vi "Insert table - 2.vi"() -> ()   [LabVIEW 2015]
uses:
  <vilib>/Platform/TimedLoop/XDataNode/timing_clust.ctl
  <vilib>/Platform/TimedLoop/XDataNode/nitl_modes.ctl
  <vilib>/Platform/TimedLoop/XDataNode/wakeup.ctl
  <vilib>/addons/database/Connection.llb/DB Tools Open Connec (Path).vi
  <vilib>/platform/TimedLoop/XDataNode/XDataNode.xnode
  <vilib>/addons/database/NI_Database_API.lvlib
  <vilib>/Platform/TimedLoop/XDataNode/XDNodeRunTimeDep.lvlib
panel:
  out "floor(x/y)":dbl
  out "Time":u32
  out "Counter":i32
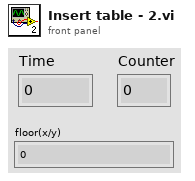
[diagram p1: front panel]
types:
  T1 = typedef "NI_Database_API.lvlib/Conn ObjectReference.ctl" = refnum<k1>
  T2 = typedef "XDNodeRunTimeDep.lvlib/timing_clust.ctl" = cluster{"Expected End [f-1]":u64, "Actual End [f-1]":u64, "Finished Late? [f-1]":bool, "Expected End [i-1]":u64, "Actual End [i-1]":u64, "Finished Late? [i-1]":bool, "Expected Start [i]":u64, "Actual Start [i]":u64, "Expected Start [f]":u64, "Actual Start [f]":u64, "Source Name":string, "Structure Name":string, "Period":i64, "Deadline":i64, "Offset":i64, "Start":i64, "Priority":i32, "Timeout":i32, "Mode":T3, "Wakeup Reason":T4, "Error":errorcluster, "Source Type":string, "Secondary Source Type":string, "Global End Time":u64, "Global Start Time":u64, "Frame Duration":u64, "Iteration Duration":u64, "Assigned CPU":i32, "I/O Scan Engine Mode":u32}
  T3 = typedef "XDNodeRunTimeDep.lvlib/nitl_modes.ctl" = enum32{"No Change", "Process missed periods, maintain original phase", "Discard missed periods, maintain original phase", "Process missed periods, ignore original phase", "Discard missed periods, ignore original phase"}
  T4 = typedef "XDNodeRunTimeDep.lvlib/wakeup.ctl" = enum32{"Normal", "Aborted", "Asynchronous wakeup", "Timing source error", "Timed loop error", "Timeout"}
  T5 = cluster{i32, i32, i32, i32, i32, i32, i32, i32, i32, i32, i32, i32, i32, i32, i32, i32, i32, i32, i32, i32, i32, i32, i32, i32, i32, i32, i32, i32, i32, i32, i32, i32, i32, i32, i32, i32, i32, i32, i32, i32, i32, i32, i32, i32, i32, i32, i32, i32, i32, i32, i32, i32, i32, i32, i32, i32, i32, i32, i32, i32, i32, i32, i32, i32, i32, i32, i32, i32, i32, i32, i32, i32, i32, i32, i32, i32, i32, i32, i32, i32, i32, i32, i32, i32, i32, i32, i32, i32, i32, i32, i32, i32, i32, i32, i32, i32, i32, i32, i32, i32}
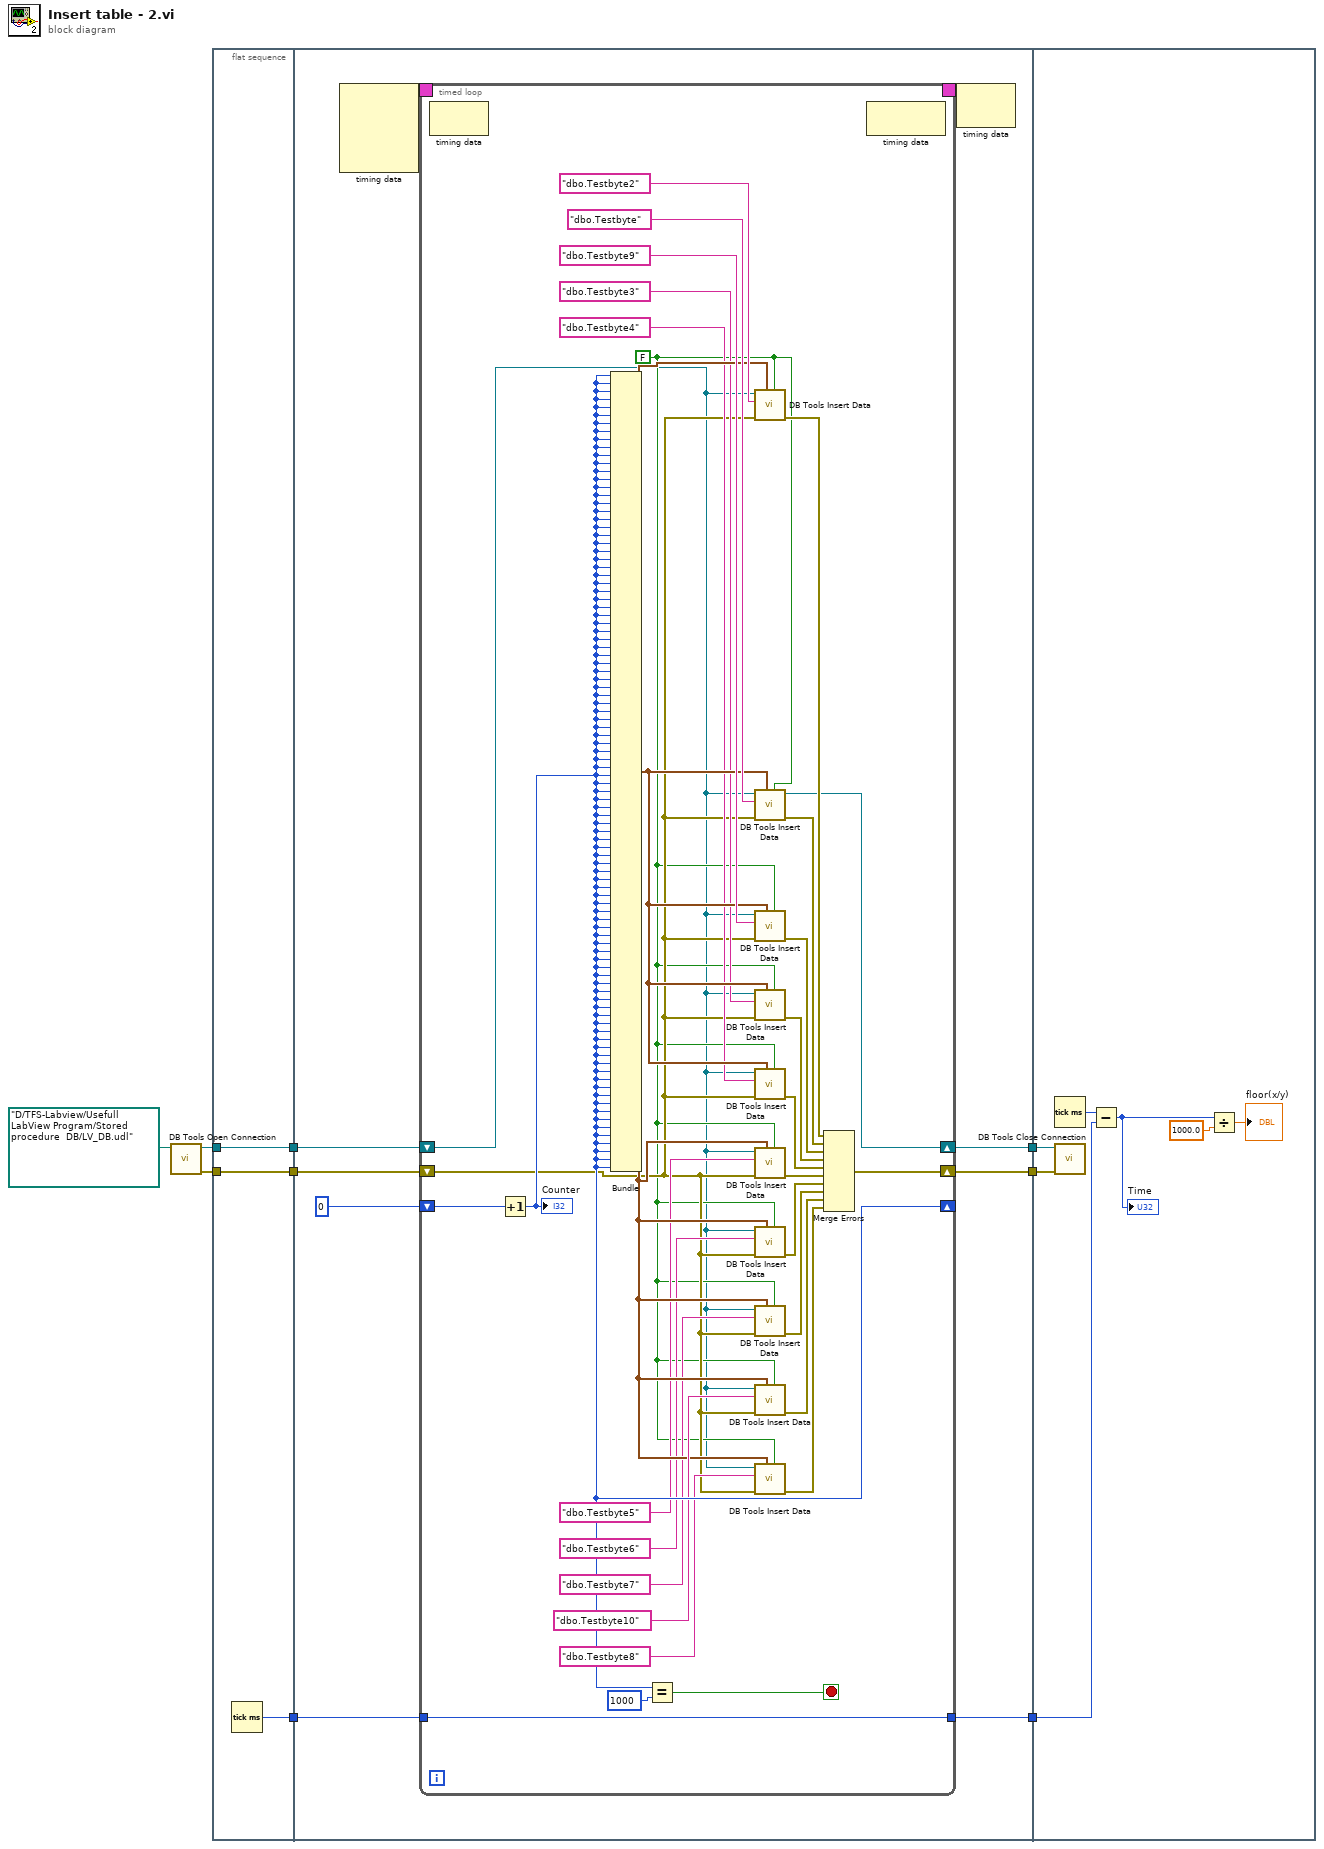
[diagram p0: block diagram]
diagram:
  n1 = call-poly <vilib>:"DB Tools Open Connection.vi"("connection information"=path "D:/TFS-Labview/Usefull LabView Program/Stored procedure  DB/LV_DB.udl") -> ("error out"=w1:errorcluster, "connection reference"=w3:T1)  [unwired: 7 in]
  n2 = flat-sequence {
    tunnel: [w12] -> w9
    tunnel: [w11] -> w8
    tunnel: w3 -> [w11]
    tunnel: [w10] -> w2
    tunnel: w1 -> [w10]
    tunnel: [w20] -> w7
    tunnel: [w18] -> w6
    tunnel: w9 -> [w19]
    tunnel: w8 -> [w17]
    tunnel: [w16] -> w5
    tunnel: w2 -> [w15]
    tunnel: w7 -> [w60]
    tunnel: w6 -> [w62]
    tunnel: w5 -> [w61]
    frame #0 {
      n3 = Tick Count (ms)() -> (millisecond timer value=w12:u32)
    }
    frame #1 {
      n4 = node-c288() -> (w14:T2)  [unwired: 4 in]
      n5 = timed-loop {
        shift-right: [w44] -> w20
        shift-left: w15 -> [w33]
        shift-right: [w43] -> _
        shift-left: 0 -> [w52]
        tunnel: [w51] -> w18
        tunnel: w19 -> [w51]
        shift-right: [w23] -> w16
        shift-left: w17 -> [w22]
        timing: w14 -> [_]
        timing-out: [_] -> w13
        stop <- w49 stop-if-true
        w24 = FALSE ("create table? (F)")
        n6 = node-c288() -> ()  [unwired: 1 in, 1 out]
        n7 = Increment(x=w52) -> (x+1=w43:i32)
        "Counter" <- w43
        n8 = Bundle(w43, w43, w43, w43, w43, w43, w43, w43, w43, w43, w43, w43, w43, w43, w43, w43, w43, w43, w43, w43, w43, w43, w43, w43, w43, w43, w43, w43, w43, w43, w43, w43, w43, w43, w43, w43, w43, w43, w43, w43, w43, w43, w43, w43, w43, w43, w43, w43, w43, w43, w43, w43, w43, w43, w43, w43, w43, w43, w43, w43, w43, w43, w43, w43, w43, w43, w43, w43, w43, w43, w43, w43, w43, w43, w43, w43, w43, w43, w43, w43, w43, w43, w43, w43, w43, w43, w43, w43, w43, w43, w43, w43, w43, w43, w43, w43, w43, w43, w43, w43) -> (w39:T5)  [unwired: 1 in]
        n9 = Equal?(x=w43, y=1000 ("Numeric")) -> (x = y?=w49:bool)
        n10 = call <vilib>:"DB Tools Insert Data.vi"("create table? (F)"=w24, "data"=w39, "error in (no error)"=w33, "table"="dbo.Testbyte2" ("SQL query"), "connection reference"=w22) -> ("error out"=w46:errorcluster)  [unwired: 5 in, 1 out]
        n11 = call <vilib>:"DB Tools Insert Data.vi"("create table? (F)"=w24, "data"=w39, "error in (no error)"=w33, "table"="dbo.Testbyte" ("SQL query"), "connection reference"=w22) -> ("error out"=w45:errorcluster, "connection reference out"=w23:T1)  [unwired: 5 in]
        n12 = call <vilib>:"DB Tools Insert Data.vi"("create table? (F)"=w24, "data"=w39, "error in (no error)"=w33, "table"="dbo.Testbyte9" ("SQL query"), "connection reference"=w22) -> ("error out"=w32:errorcluster)  [unwired: 5 in, 1 out]
        n13 = call <vilib>:"DB Tools Insert Data.vi"("create table? (F)"=w24, "data"=w39, "error in (no error)"=w33, "table"="dbo.Testbyte3" ("SQL query"), "connection reference"=w22) -> ("error out"=w31:errorcluster)  [unwired: 5 in, 1 out]
        n14 = call <vilib>:"DB Tools Insert Data.vi"("create table? (F)"=w24, "data"=w39, "error in (no error)"=w33, "table"="dbo.Testbyte4" ("SQL query"), "connection reference"=w22) -> ("error out"=w30:errorcluster)  [unwired: 5 in, 1 out]
        n15 = call <vilib>:"DB Tools Insert Data.vi"("create table? (F)"=w24, "data"=w39, "error in (no error)"=w33, "table"="dbo.Testbyte5" ("SQL query"), "connection reference"=w22) -> ("error out"=w29:errorcluster)  [unwired: 5 in, 1 out]
        n16 = call <vilib>:"DB Tools Insert Data.vi"("create table? (F)"=w24, "data"=w39, "error in (no error)"=w33, "table"="dbo.Testbyte6" ("SQL query"), "connection reference"=w22) -> ("error out"=w28:errorcluster)  [unwired: 5 in, 1 out]
        n17 = call <vilib>:"DB Tools Insert Data.vi"("create table? (F)"=w24, "data"=w39, "error in (no error)"=w33, "table"="dbo.Testbyte7" ("SQL query"), "connection reference"=w22) -> ("error out"=w27:errorcluster)  [unwired: 5 in, 1 out]
        n18 = call <vilib>:"DB Tools Insert Data.vi"("create table? (F)"=w24, "data"=w39, "error in (no error)"=w33, "table"="dbo.Testbyte10" ("SQL query"), "connection reference"=w22) -> ("error out"=w26:errorcluster)  [unwired: 5 in, 1 out]
        n19 = call <vilib>:"DB Tools Insert Data.vi"("create table? (F)"=w24, "data"=w39, "error in (no error)"=w33, "table"="dbo.Testbyte8" ("SQL query"), "connection reference"=w22) -> ("error out"=w25:errorcluster)  [unwired: 5 in, 1 out]
        n20 = Merge Errors(w46, w45, w32, w31, w30, w29, w28, w27, w26, w25) -> (w44:errorcluster)
        n21 = node-c288() -> ()  [unwired: 1 in, 1 out]
      }
      n22 = node-c288(w13) -> ()  [unwired: 1 out]
    }
    frame #2 {
      n23 = Tick Count (ms)() -> (millisecond timer value=w63:u32)
      n24 = call <vilib>:"DB Tools Close Connection.vi"("error in (no error)"=w60, "connection reference"=w61) -> ()  [unwired: 5 in, 1 out]
      n25 = Subtract(x=w63, y=w62) -> (x-y=w57:u32)
      "Time" <- w57
      n26 = Divide(x=w57, y=1000.0) -> (x/y=→"floor(x/y)":dbl)
    }
  }
